vi "RVC 5-link serial robot with tool and more stuff.vi"() -> ()   [LabVIEW 2013]
uses:
  <vilib>/robotics/Kinematics/Robot/Robot Pose.ctl
  <vilib>/Analysis/baseanly.llb/Real A x B.vi
  <vilib>/Analysis/_algsub.llb/Vector Norm.vi
  <vilib>/Analysis/_algsub.llb/Real Vector Norm.vi
  <vilib>/Analysis/baseanly.llb/Outer Product.vi
  <vilib>/Analysis/baseanly.llb/Real Outer Product.vi
  <vilib>/robotics/Kinematics/Create Lie Group Matrix.vi
  <vilib>/robotics/Kinematics/Analytical/Initialize Generic Serial Arm.vi
  <vilib>/Analysis/7linalg.llb/Create Special Matrix.vi
  <vilib>/Analysis/7linalg.llb/Create Special Real Matrix.vi
  <vilib>/Analysis/Matrix/Numeric/Multiply/Multiply.vi
  <vilib>/Analysis/Matrix/Numeric/Multiply/Multiply - RM,R.vi
  <vilib>/Analysis/Matrix/Numeric/Multiply/Multiply - R,RM.vi
  <vilib>/Analysis/Matrix/Numeric/Add/Add.vi
  <vilib>/Analysis/Matrix/Numeric/Add/Add - RM,RM.vi
  <vilib>/robotics/Kinematics/Analytical/NI_Robotics_AnalyticKinematics.lvlib
  <vilib>/robotics/Kinematics/Link/Joint Type.ctl
  <vilib>/robotics/Kinematics/Link/NI_Robotics_Link.lvclass
  <vilib>/robotics/Kinematics/Robot/NI_Robotics_Serial Robot Arm.lvclass
  <vilib>/robotics/Kinematics/NI_Kinematics.lvlib
  <vilib>/Analysis/NI_AALBase.lvlib
panel:
  in  "Ring":u16(ring) items=["Origin", "Above", "Up-side down"]
  in  "End-Effector Offcenter":bool
  out "transformation":picture
  in  "Pose":u16(ring) items=["qz", "qr", "qs", "qn"]
  in  "stop":bool
  out "3D Picture":refnum<vi>(3d-picture)
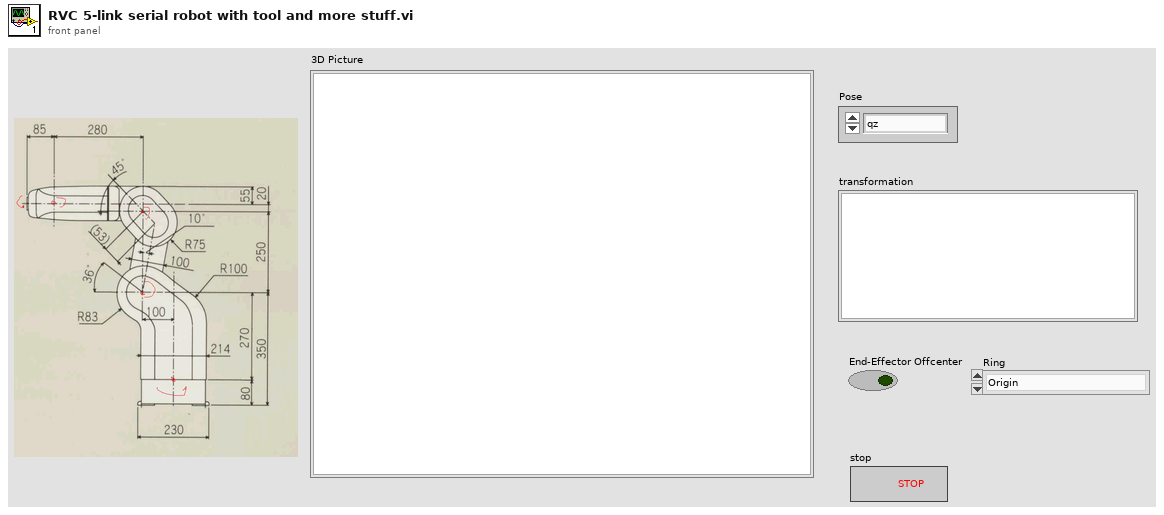
[diagram p1: front panel]
types:
  T1 = typedef "NI_Robotics_Serial Robot Arm.lvclass/Robot Pose.ctl" = cluster{"name":string, "description":string, "joint positions":dbl[]}
  T2 = typedef "NI_Robotics_Link.lvclass/Joint Type.ctl" = enum16{"Revolute", "Prismatic"}
  T3 = cluster{"Twist Angle":dbl, "Length":dbl, "Rotation Angle":dbl, "Offset Distance":dbl, "Joint Type":T2, "Joint Coordinate Offset":dbl}[]
  T4 = typedef "DH Kinematic Parameters.ctl" = cluster{"twist angle":dbl, "length":dbl, "rotation angle":dbl, "offset distance":dbl, "joint type":T2, "joint coordinate offset":dbl}
  T5 = typedef "NI_Matrix.lvlib/RealMatrix.ctl" = dbl[][]
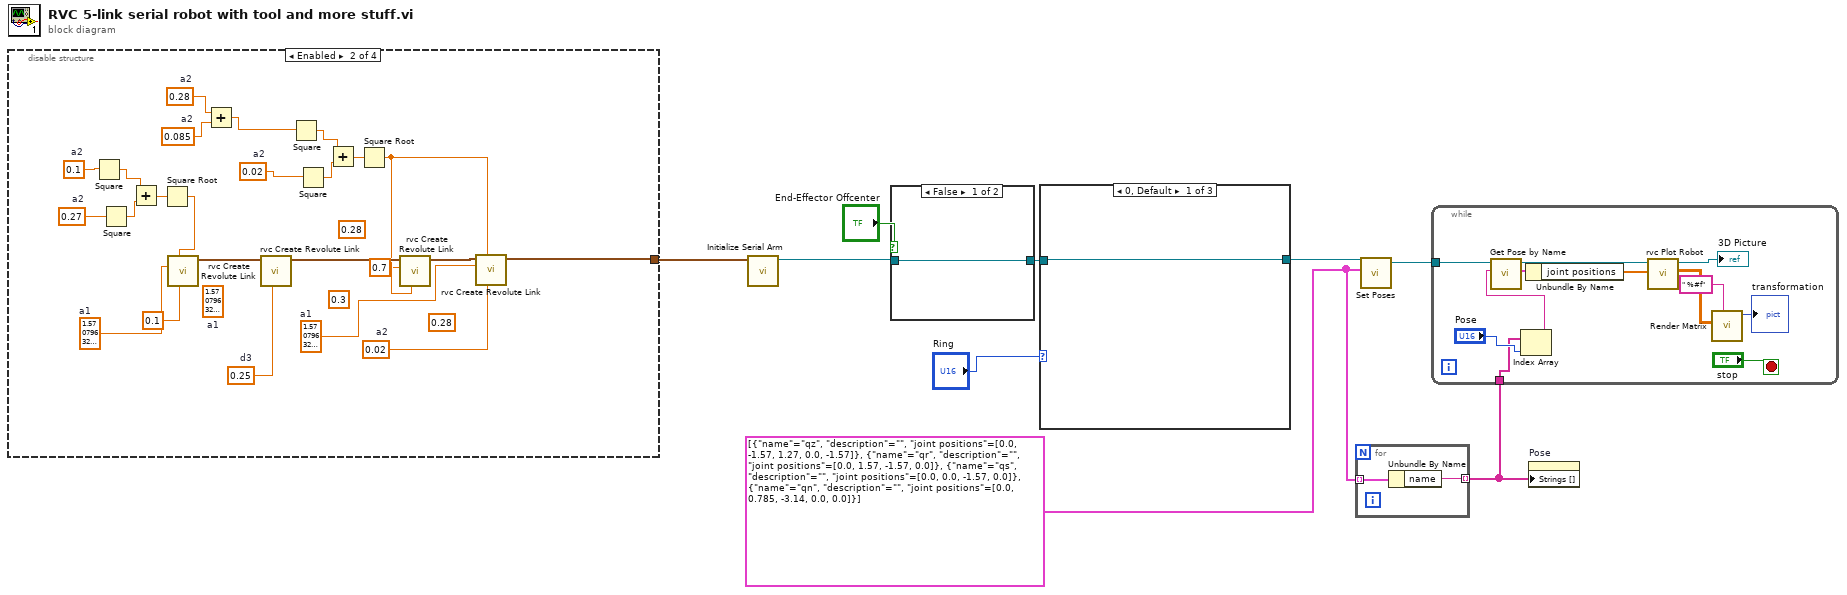
[diagram p0: block diagram]
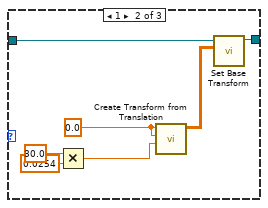
[diagram p2: hidden frame]
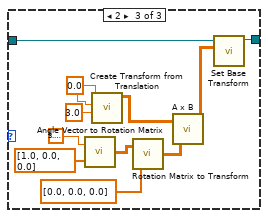
[diagram p3: hidden frame]
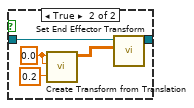
[diagram p4: hidden frame]
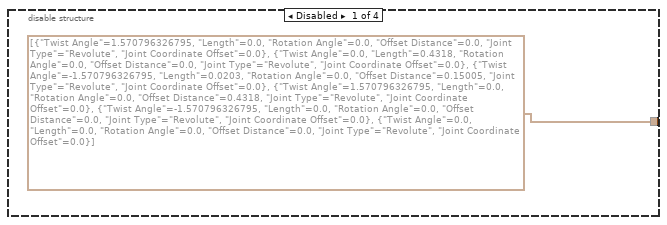
[diagram p5: hidden frame]
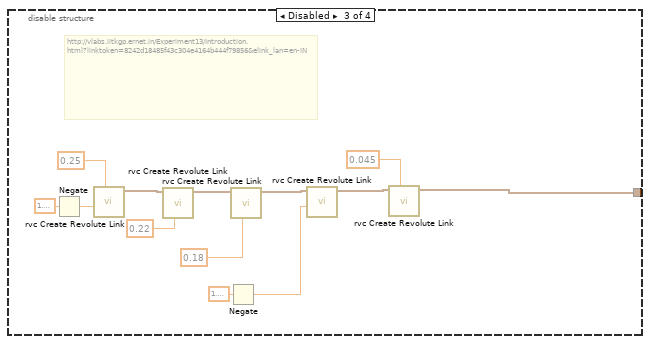
[diagram p6: hidden frame]
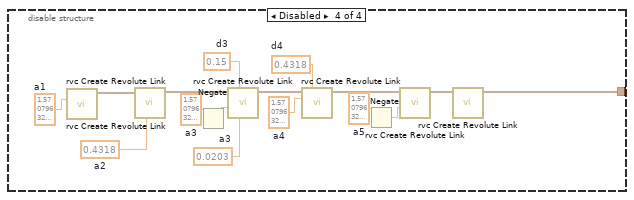
[diagram p7: hidden frame]
diagram:
  w7 = T1[] [{"name"="qz", "description"="", "joint positions"=[0.0, -1.57, 1.27, 0.0, -1.57]}, {"name"="qr", "description"="", "joint positions"=[0.0, 1.57, -1.57, 0.0]}, {"name"="qs", "description"="", "joint positions"=[0.0, 0.0, -1.57, 0.0]}, {"name"="qn", "description"="", "joint positions"=[0.0, 0.785, -3.14, 0.0, 0.0]}] ("serial arm poses")
  n1 = disable-structure shown="Enabled" {
    disable-tunnel: [T3 [{"Twist Angle"=1.570796326795, "Length"=0.0, "Rotation Angle"=0.0, "Offset Distance"=0.0, "Joint Type"=enum."Revolute", "Joint Coordinate Offset"=0.0}, {"Twist Angle"=0.0, "Length"=0.4318, "Rotation Angle"=0.0, "Offset Distance"=0.0, "Joint Type"=enum."Revolute", "Joint Coordinate Offset"=0.0}, {"Twist Angle"=-1.570796326795, "Length"=0.0203, "Rotation Angle"=0.0, "Offset Distance"=0.15005, "Joint Type"=enum."Revolute", "Joint Coordinate Offset"=0.0}, {"Twist Angle"=1.570796326795, "Length"=0.0, "Rotation Angle"=0.0, "Offset Distance"=0.4318, "Joint Type"=enum."Revolute", "Joint Coordinate Offset"=0.0}, {"Twist Angle"=-1.570796326795, "Length"=0.0, "Rotation Angle"=0.0, "Offset Distance"=0.0, "Joint Type"=enum."Revolute", "Joint Coordinate Offset"=0.0}, {"Twist Angle"=0.0, "Length"=0.0, "Rotation Angle"=0.0, "Offset Distance"=0.0, "Joint Type"=enum."Revolute", "Joint Coordinate Offset"=0.0}] w19 w36 w62] -> w9
    frame Disabled {
    }
    frame Enabled {
      (unwired) 0.28 ("length (a)")
      (unwired) 0.3 ("offset distance (d)")
      (unwired) 1.5707963267948966  # a1
      w14 = 0.02  # a2
      w15 = 0.02  # a2
      w18 = 0.085  # a2
      w11 = 1.5707963267948966  # a1
      w17 = 0.28  # a2
      w30 = 0.27  # a2
      (unwired) 0.28 ("length (a)")
      w24 = 1.5707963267948966  # a1
      w32 = 0.25  # d3
      w31 = 0.1  # a2
      n2 = Square(x=w31) -> (x^2=w28:dbl)
      n3 = Square(x=w30) -> (x^2=w29:dbl)
      n4 = Add(x=w28, y=w29) -> (x+y=w27:dbl)
      n5 = Square Root(x=w27) -> (sqrt(x)=w26:dbl)
      n6 = call "rvc Create Revolute Link.vi"("length (a)"=0.1 ("offset distance (d)"), "offset distance (d)"=w26, "twist angle (alpha)"=w24) -> ("Array"=w34:T4[])  [unwired: 8 in]
      n7 = Add(x=w17, y=w18) -> (x+y=w16:dbl)
      n8 = call "rvc Create Revolute Link.vi"("length (a)"=w32, "Array 2"=w34) -> ("Array"=w33:T4[])  [unwired: 9 in]
      n9 = Square(x=w16) -> (x^2=w22:dbl)
      n10 = Square(x=w15) -> (x^2=w21:dbl)
      n11 = Add(x=w22, y=w21) -> (x+y=w23:dbl)
      n12 = Square Root(x=w23) -> (sqrt(x)=w13:dbl)
      n13 = call "rvc Create Revolute Link.vi"("length (a)"=w13, "rotation angle (theta)"=0.7, "Array 2"=w33) -> ("Array"=w20:T4[])  [unwired: 8 in]
      n14 = call "rvc Create Revolute Link.vi"("length (a)"=w14, "offset distance (d)"=w13, "twist angle (alpha)"=w11, "Array 2"=w20) -> ("Array"=w19:T4[])  [unwired: 7 in]
    }
    frame Disabled {
      # "http://vlabs.iitkgp.ernet.in/Experiment13/Introduction.html?linktoken=8242d18485f43c304e4164b444f79856&elink_lan=en-IN"
      n15 = Negate(x=1.5707963267948966 ("twist angle (alpha)")) -> (-x=w46:dbl)
      n16 = call "rvc Create Revolute Link.vi"("offset distance (d)"=0.25, "twist angle (alpha)"=w46) -> ("Array"=w44:T4[])  [unwired: 9 in]
      n17 = call "rvc Create Revolute Link.vi"("length (a)"=0.22, "Array 2"=w44) -> ("Array"=w42:T4[])  [unwired: 9 in]
      n18 = Negate(x=1.5707963267948966 ("twist angle (alpha)")) -> (-x=w38:dbl)
      n19 = call "rvc Create Revolute Link.vi"("length (a)"=0.18, "Array 2"=w42) -> ("Array"=w40:T4[])  [unwired: 9 in]
      n20 = call "rvc Create Revolute Link.vi"("twist angle (alpha)"=w38, "Array 2"=w40) -> ("Array"=w37:T4[])  [unwired: 9 in]
      n21 = call "rvc Create Revolute Link.vi"("offset distance (d)"=0.045, "Array 2"=w37) -> ("Array"=w36:T4[])  [unwired: 9 in]
    }
    frame Disabled {
      w49 = 1.5707963267948966  # a5
      w50 = 0.4318  # d4
      w51 = 1.5707963267948966  # a4
      w53 = 1.5707963267948966  # a3
      w54 = 0.15  # d3
      w55 = 0.0203  # a3
      w59 = 0.4318  # a2
      w61 = 1.5707963267948966  # a1
      n22 = call "rvc Create Revolute Link.vi"("twist angle (alpha)"=w61) -> ("Array"=w60:T4[])  [unwired: 10 in]
      n23 = call "rvc Create Revolute Link.vi"("length (a)"=w59, "Array 2"=w60) -> ("Array"=w58:T4[])  [unwired: 9 in]
      n24 = Negate(x=w53) -> (-x=w52:dbl)
      n25 = call "rvc Create Revolute Link.vi"("length (a)"=w55, "offset distance (d)"=w54, "twist angle (alpha)"=w52, "Array 2"=w58) -> ("Array"=w57:T4[])  [unwired: 7 in]
      n26 = call "rvc Create Revolute Link.vi"("offset distance (d)"=w50, "twist angle (alpha)"=w51, "Array 2"=w57) -> ("Array"=w56:T4[])  [unwired: 8 in]
      n27 = Negate(x=w49) -> (-x=w48:dbl)
      n28 = call "rvc Create Revolute Link.vi"("twist angle (alpha)"=w48, "Array 2"=w56) -> ("Array"=w63:T4[])  [unwired: 9 in]
      n29 = call "rvc Create Revolute Link.vi"("Array 2"=w63) -> ("Array"=w62:T4[])  [unwired: 10 in]
    }
  }
  n30 = call-poly <vilib>:"Initialize Serial Arm.vi"("kinematic parameters"=w9) -> ("serial arm out"=w5:refnum<class "NI_Robotics_Serial Robot Arm.lvclass">)  [unwired: 9 in, 1 out]
  n31 = case shown="False" "End-Effector Offcenter" {
    tunnel: w5 -> [w64 w69]
    tunnel: [w64 w65] -> w4
    frame False {
    }
    frame True {
      w66 = 0.0 ("x")
      n32 = call <vilib>:"Create Transform from Translation.vi"("z"=0.2, "y"=w66, "x"=w66) -> ("transform"=w68:T5)  [unwired: 8 in]
      n33 = call <vilib>:"Set End Effector Transform.vi"("end effector transform"=w68, "serial arm in"=w69) -> ("serial arm out"=w65:refnum<class "NI_Robotics_Serial Robot Arm.lvclass">)  [unwired: 8 in, 1 out]
    }
  }
  n34 = case shown="0, Default" "Ring" {
    tunnel: w4 -> [w70 w77 w88]
    tunnel: [w70 w76 w87] -> w3
    frame 0, Default {
    }
    frame 1 {
      w74 = 0.0 ("x")
      n35 = Multiply(x=30.0, y=0.0254) -> (x*y=w73:dbl)
      n36 = call <vilib>:"Create Transform from Translation.vi"("z"=w73, "y"=w74, "x"=w74) -> ("transform"=w75:T5)  [unwired: 8 in]
      n37 = call <vilib>:"Set Base Transform.vi"("base transform"=w75, "serial arm in"=w77) -> ("serial arm out"=w76:refnum<class "NI_Robotics_Serial Robot Arm.lvclass">)  [unwired: 8 in, 1 out]
    }
    frame 2 {
      w84 = 0.0 ("z")
      n38 = call <vilib>:"Angle Vector to Rotation Matrix.vi"("vector"=dbl[] [1.0, 0.0, 0.0], "angle"=3.141592653589793) -> ("rotation matrix"=w80:T5)
      n39 = call <vilib>:"Create Transform from Translation.vi"("z"=3.0, "y"=w84, "x"=w84) -> ("transform"=w85:T5)  [unwired: 8 in]
      n40 = call <vilib>:"Rotation Matrix to Transform.vi"("translation vector"=dbl[] [0.0, 0.0, 0.0], "rotation matrix"=w80) -> ("transform"=w79:T5)
      n41 = call-poly <vilib>:"A x B.vi"("B"=w79, "A"=w85) -> ("A x B"=w86:T5)  [unwired: 1 out]
      n42 = call <vilib>:"Set Base Transform.vi"("base transform"=w86, "serial arm in"=w88) -> ("serial arm out"=w87:refnum<class "NI_Robotics_Serial Robot Arm.lvclass">)  [unwired: 8 in, 1 out]
    }
  }
  n43 = for {
    tunnel: w7 -> [w90] mode=indexing
    tunnel: [w89] -> w6 mode=indexing
    n44 = Unbundle By Name(w90) -> ("name"=w89:string)
  }
  n45 = call <vilib>:"Set Poses.vi"("serial arm poses"=w7, "serial arm in"=w3) -> ("serial arm out"=w8:refnum<class "NI_Robotics_Serial Robot Arm.lvclass">)  [unwired: 8 in, 1 out]
  n46 = while {
    tunnel: w8 -> [w99]
    tunnel: w6 -> [w95]
    stop <- "stop" stop-if-true
    n47 = Index Array(array=w95, index="Pose") -> (element=w94:string)
    n48 = call <vilib>:"Get Pose by Name.vi"("name"=w94, "serial arm in"=w99) -> ("serial arm pose"=w101:T1, "serial arm out"=w98:refnum<class "NI_Robotics_Serial Robot Arm.lvclass">)  [unwired: 7 in, 1 out]
    n49 = Unbundle By Name(w101) -> ("joint positions"=w100:dbl[])
    n50 = call "rvc Plot Robot.vi"("joint positions"=w100, "NI_Robotics_Serial Robot Arm in"=w98) -> ("forward kinematics"=w93:T5, "Scene Object Out"=→"3D Picture":refnum<vi>)  [unwired: 8 in]
    n51 = call "Render Matrix.vi"("format string"=" %#f", "A"=w93) -> ("picture out"=→"transformation":picture)  [unwired: 9 in]
  }
  n52 = property on="Pose" class="Ring (strict)"("Strings []"=w6) -> ()  [unwired: 2 in, 2 out]
